vi "getWfFromShwfsFile.vi"(8 "error in (no error)":errorcluster, 10 "Wfs Err Data":path=path "/home/ttsai/Documents/stash/ts_tcs_ofc/testData/shwfs_wfs_error.txt", 11 "OptStateEsti in":refnum<class "OptStateEsti.lvclass">) -> (0 "error out":errorcluster, 1 "Sensor Name":string[](array[string])=["R:4,4 S:0,0", "R:0,4 S:2,0", "R:0,0 S:2,2", "R:4,0 S:0,2"], 2 "Wavefront Error":dbl[][](array[numeric]), 3 "OptStateEsti out":refnum<class "OptStateEsti.lvclass">)   [LabVIEW 2016, in "OfcFunc.lvlib" / "OptStateEsti.lvclass"]
doc: "Get the wavefront error from the SHWFS file."
uses:
  OptStateEsti.lvclass
  MatOper/getSubArray2D.vi
  MatOper/MatOper.lvclass
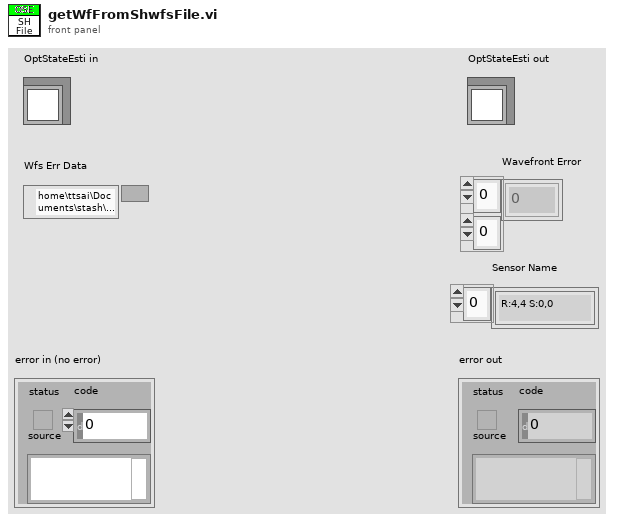
[diagram p1: front panel]
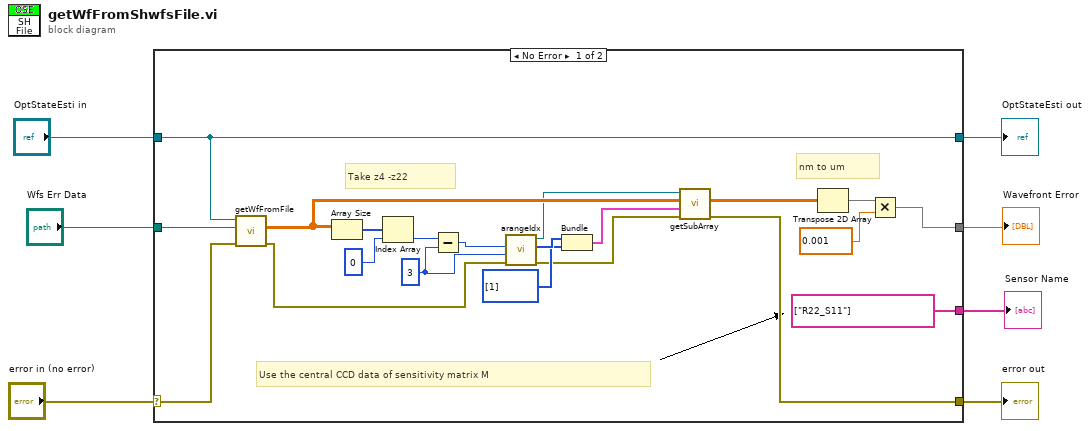
[diagram p0: block diagram]
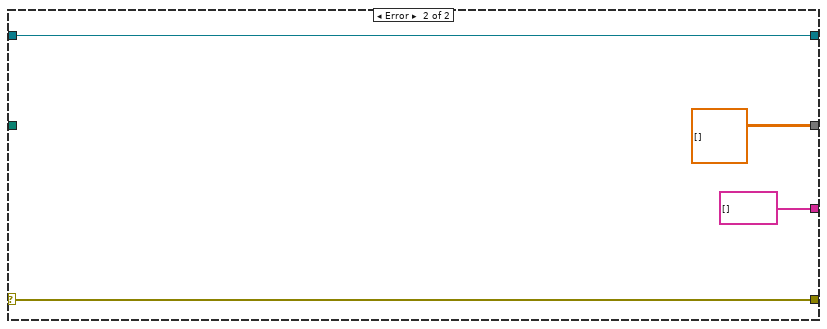
[diagram p2: hidden frame]
diagram:
  n1 = case shown="No Error" "error in (no error)" {
    selector: "error in (no error)" -> [w26 w32]
    tunnel: [w12 w32] -> w6
    tunnel: [w28 w31] -> w4
    tunnel: "OptStateEsti in" -> [w28 w31]
    tunnel: "Wfs Err Data" -> [w27 _]
    tunnel: [string[] ["R22_S11"] ("Sensor Name") string[] [] ("Sensor Name")] -> w1
    tunnel: [w13 dbl[][] [] ("Wavefront Error")] -> w2
    frame No Error {
      w14 = 3 ("index")
      # "Use the central CCD data of sensitivity matrix M"
      # "Take z4 -z22"
      # "nm to um"
      n2 = call "getWfFromFile.vi"("error in (no error)"=w26, "Wfs Err Data"=w27, "OptStateEsti in"=w28) -> ("error out"=w9:errorcluster, "Wavefront Error"=w23:dbl[][])  [unwired: 5 in, 2 out]
      n3 = Array Size(array=w23) -> (size(s)=w25:i32[])
      n4 = Index Array(array=w25, index=0) -> (element=w16:i32)
      n5 = Subtract(x=w16, y=w14) -> (x-y=w15:i32)
      n6 = call "arangeIdx.vi"("error in (no error)"=w9, "Offset"=w14, "Number"=w15) -> ("error out"=w8:errorcluster, "Idx Array"=w22:i32[], "MatOper out"=w10:refnum<class "MatOper.lvclass">)  [unwired: 6 in]
      n7 = Bundle("Idx Array"=w22, i32[] [1]) -> (w20:cluster{"Idx Array":i32[], i32[]})  [unwired: 1 in]
      n8 = call-poly "getSubArray.vi"("error in (no error)"=w8, "Index Array Cluster"=w20, "2D Array"=w23, "MatOper in"=w10) -> ("error out"=w12:errorcluster, "Sub-Array"=w19:dbl[][])  [unwired: 5 in, 1 out]
      n9 = Transpose 2D Array(2D array=w19) -> (transposed array=w18:dbl[][])
      n10 = Multiply(x=w18, y=0.001) -> (x*y=w13:dbl[][])
    }
    frame Error {
    }
  }
  "error out" <- w6
  "OptStateEsti out" <- w4
  "Wavefront Error" <- w2
  "Sensor Name" <- w1
